vi "Read_Exposures.vi"(6 "ref in":i32, 7 "sequencer":T1(array[cluster]), 8 "error in":errorcluster) -> (0 "ref out":i32, 1 "ROI":T2, 2 "loaded images":u16[][][](array[numeric]), 4 "computations":T3(array[cluster]), 5 "error out":errorcluster)   [LabVIEW 2010]
uses:
  <userlib>/bias2/subvis/ROI_rect.ctl
  <vilib>/addons/h5labview2/attrib/H5Aread.llb/H5Aread.xnode
  <vilib>/addons/h5labview2/dataset/H5Dread.llb/H5Dread.xnode
  <vilib>/addons/h5labview2/base/H5Equery.vi
  <vilib>/addons/h5labview2/h5labview.lib
  <vilib>/addons/h5labview2/group/H5G.lvlib
  <vilib>/addons/h5labview2/type/H5T.lvlib
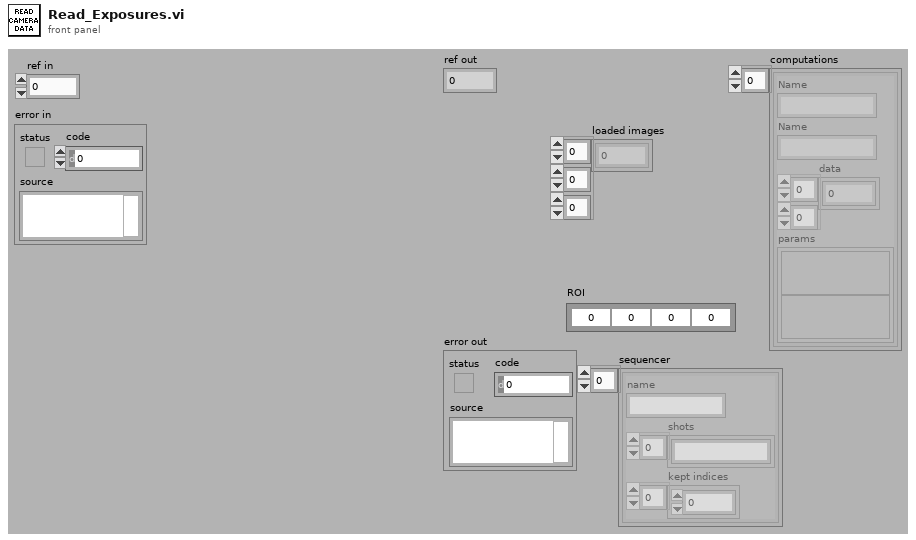
[diagram p1: front panel]
types:
  T1 = cluster{"name":string, "shots":string[], "kept indices":i32[]}[]
  T2 = typedef "ROI_rect.ctl" = cluster{"left":i32, "top":i32, "right":i32, "bottom":i32}
  T3 = cluster{"Name":string, "Name":string, "data":sgl[][], "params":variant[]}[]
  T4 = cluster{"name":string, "shots":string[], "kept indices":i32[]}
  T5 = typedef "hid_t.ctl" = i32
  T6 = typedef "h5o_type.ctl" = enum16{"Group", "Dataset", "Named type"}
  T7 = typedef "hclass_t.ctl" = enum16{"H5T_INTEGER", "H5T_FLOAT", "H5T_TIME", "H5T_STRING", "H5T_BITFIELD", "H5T_OPAQUE", "H5T_COMPOUND", "H5T_REFERENCE", "H5T_ENUM", "H5T_VLEN", "H5T_ARRAY"}
  T8 = cluster{"name":string, "name":string, "data":sgl[][], variant[]}
  T9 = cluster{"name":string, "name":string, "data":sgl[][], "params":variant[]}[]
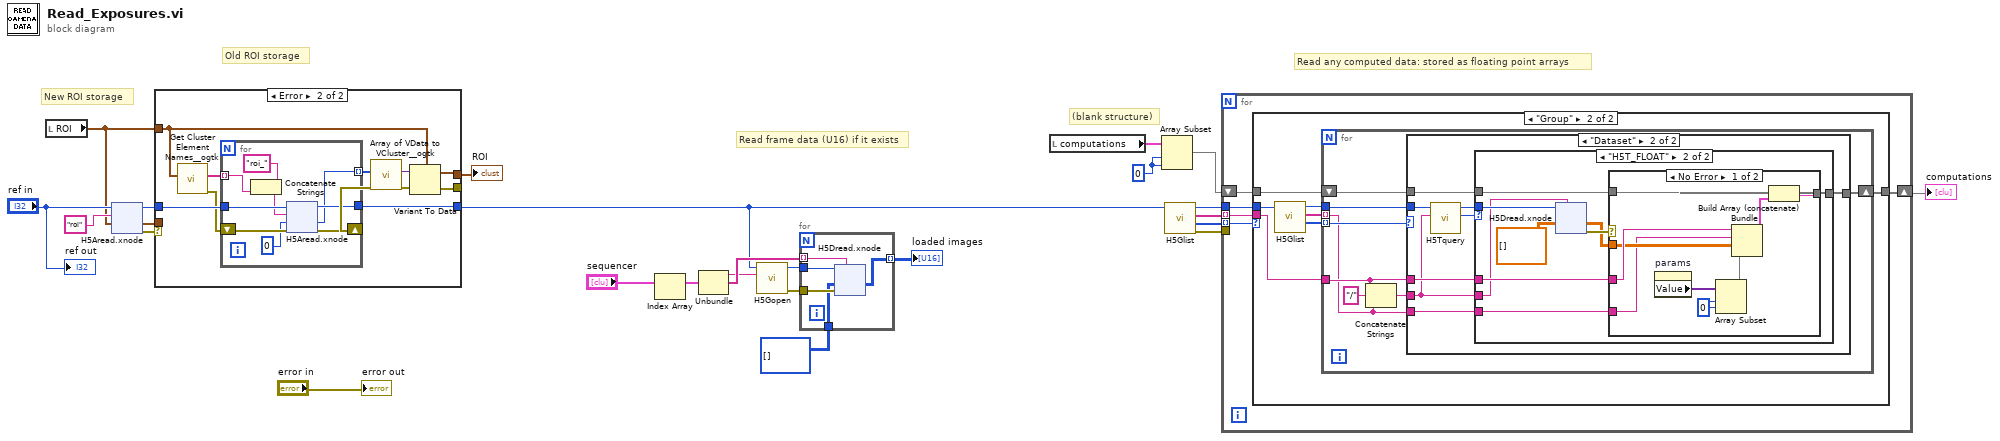
[diagram p0: block diagram]
diagram:
  w23 = 0 ("length")
  # "(blank structure)"
  # "Old ROI storage"
  # "New ROI storage"
  # "Read any computed data: stored as floating point arrays"
  # "Read frame data (U16) if it exists"
  n1 = local read "ROI"() -> (w12:T2)
  n2 = xnode "H5Aread.xnode"("default"=w12, "attrib name"="roi" ("prefix"), "ref in"="ref in") -> ("error out"=w10:errorcluster, "data"=w11:T2, "ref out"=w14:i32)  [unwired: 3 in, 1 out]
  n3 = case shown="Error" w10 {
    tunnel: w12 -> [_ w34]
    tunnel: w14 -> [w26 w37]
    tunnel: w11 -> [w27 _]
    tunnel: [w27 w29] -> w21
    tunnel: [w26 w36] -> w5
    tunnel: [_ w28] -> _
    frame No Error {
    }
    frame Error {
      n4 = call <userlib>:"Get Cluster Element Names__ogtk.vi"("Cluster"=w34) -> ("error out"=w35:errorcluster, "Element Names"=w38:string[])  [unwired: 9 in]
      n5 = for {
        tunnel: w38 -> [w46] mode=indexing
        tunnel: w37 -> [w45]
        tunnel: [w41] -> w36
        shift-right: [w42] -> w32
        shift-left: w35 -> [w44]
        tunnel: [w39] -> w33 mode=indexing
        n6 = Concatenate Strings("roi_" ("prefix"), w46) -> (w43:string)
        n7 = xnode "H5Aread.xnode"("error in (no error)"=w44, "default"=0, "attrib name"=w43, "ref in"=w45) -> ("error out"=w42:errorcluster, "data"=w39:i32, "ref out"=w41:i32)  [unwired: 2 in, 1 out]
      }
      n8 = call <userlib>:"Array of VData to VCluster__ogtk.vi"("error in (no error)"=w32, "Array"=w33) -> ("error out"=w31:errorcluster, "VCluster"=w30:variant)  [unwired: 8 in]
      n9 = Variant To Data(error in=w31, Variant=w30, type=w34) -> (error out=w28:errorcluster, data=w29:T2)
    }
  }
  "ROI" <- w21
  n10 = Index Array(array="sequencer") -> (element=w17:T4)  [unwired: 1 in]
  n11 = Unbundle(w17) -> ("name"=w6:string, "shots"=w18:string[])  [unwired: 1 out]
  n12 = call <vilib>:"H5Gopen.vi"("name"=w6, "ref in"=w5) -> ("error out"=w7:errorcluster, "group out"=w8:T5)  [unwired: 5 in]
  n13 = for {
    tunnel: w8 -> [w66]
    tunnel: w18 -> [w64] mode=indexing
    tunnel: w7 -> [w65]
    tunnel: [w62] -> w16 mode=indexing
    tunnel: u16[][] [] -> [w63]
    n14 = xnode "H5Dread.xnode"("dataset name (this)"=w64, "error in (no error)"=w65, "default"=w63, "ref in"=w66) -> ("data"=w62:u16[][])  [unwired: 2 in, 3 out]
  }
  "loaded images" <- w16
  n15 = local read "computations"() -> (w24:T3)
  n16 = Array Subset(array=w24, index=w23, length=w23) -> (w22:T3)
  n17 = call <vilib>:"H5Glist.vi"("ref in"=w5) -> ("error out"=w1:errorcluster, "types"=w2:T6[], "names"=w3:string[], "ref out"=w4:T5)  [unwired: 3 in]
  n18 = for {
    shift-right: [w84] -> w25
    shift-left: w22 -> [w85]
    tunnel: w4 -> [w82]
    tunnel: w3 -> [w81] mode=indexing
    tunnel: w2 -> [w83] mode=indexing
    tunnel: w1 -> [_]
    n19 = case shown="\"Group\"" w83 {
      tunnel: w85 -> [w86 w93]
      tunnel: [w86 w92] -> w84
      tunnel: w82 -> [_ w90]
      tunnel: w81 -> [_ w91]
      frame Default {
      }
      frame "Group" {
        n20 = call <vilib>:"H5Glist.vi"("ref in"=w90) -> ("types"=w87:T6[], "names"=w88:string[], "ref out"=w89:T5)  [unwired: 3 in, 1 out]
        n21 = for {
          shift-right: [w100] -> w92
          shift-left: w93 -> [w101]
          tunnel: w89 -> [w94]
          tunnel: w88 -> [w96] mode=indexing
          tunnel: w87 -> [w99] mode=indexing
          tunnel: w91 -> [w97]
          n22 = Concatenate Strings(w97, "/" ("string"), w96) -> (w95:string)
          n23 = case shown="\"Dataset\"" w99 {
            tunnel: w101 -> [w102 w110]
            tunnel: [w102 w109] -> w100
            tunnel: w97 -> [_ w107]
            tunnel: w96 -> [_ w108]
            tunnel: w95 -> [_ w106]
            tunnel: w94 -> [_ w105]
            frame Default {
            }
            frame "Dataset" {
              n24 = call <vilib>:"H5Tquery.vi"("obj name"=w106, "ref in"=w105) -> ("class"=w103:T7, "ref out"=w104:T5)  [unwired: 4 in, 3 out]
              n25 = case shown="\"H5T_FLOAT\"" w103 {
                tunnel: w110 -> [w111 w120]
                tunnel: [w111 w119] -> w109
                tunnel: w107 -> [_ w118]
                tunnel: w104 -> [_ w115]
                tunnel: w108 -> [_ w117]
                tunnel: w106 -> [_ w114]
                frame Default {
                }
                frame "H5T_FLOAT" {
                  n26 = xnode "H5Dread.xnode"("dataset name (this)"=w114, "default"=sgl[][] [], "ref in"=w115) -> ("error out"=w116:errorcluster, "data"=w112:sgl[][])  [unwired: 3 in, 2 out]
                  n27 = case shown="No Error" w116 {
                    tunnel: w120 -> [w143 w144]
                    tunnel: [w142 w144] -> w119
                    tunnel: w112 -> [w137 _]
                    tunnel: w118 -> [w138 _]
                    tunnel: w117 -> [w136 _]
                    frame No Error {
                      w139 = 0 ("length")
                      n28 = property on="params" class="Arr (strict)"() -> ("Value"=w141:variant[])  [unwired: 2 in, 2 out]
                      n29 = Array Subset(array=w141, index=w139, length=w139) -> (w140:variant[])
                      n30 = Bundle("name"=w138, "name"=w136, "data"=w137, w140) -> (w135:T8)  [unwired: 1 in]
                      n31 = Build Array (concatenate)(w143, w135) -> (w142:T9)
                    }
                    frame Error {
                    }
                  }
                }
              }
            }
          }
        }
      }
    }
  }
  "computations" <- w25
  "error out" <- "error in"
  "ref out" <- "ref in"
